vi "Dipper Fridge Resistance Measurement 1.0.vi"() -> ()   [LabVIEW 2011]
uses:
  <vilib>/express/express arith-compare/Formula/XNode/ExpressFormulaBlockNode.xnode
panel:
  out "Heater Power (%)":string
  in  "Save":bool
  out "var":i32
  in  "error in (no error) 2":errorcluster
  in  "Output Range":string(combo)
  in  "Heater Power (%)":dbl caption="y"
  out "Heater Type (in Ohm)":string
  out "Heater Current (in %)":string
  out "Heater":bool
  in  "Heater":bool
  out "x+y":dbl
  out "Boolean":bool
  in  "Power":bool
  in  "Date format (0)":enum16{"short", "long", "abbreviated"}(ring)
  out "Lakeshore":cluster{dbl[], dbl[unit][]}(graph)
  out "Chanel B":cluster{dbl[], dbl[unit][]}(graph)
  out "size (in bytes)":i64
  out "Chanel A":cluster{dbl[], dbl[]}(graph)
  out "Warning":string="Can't be smaller than 1 s"
  in  "File Path":path
  out "current time":timestamp
  out "Number of Data points":i32
  in  "Time delay":u32
  in  "error in (no error)":errorcluster
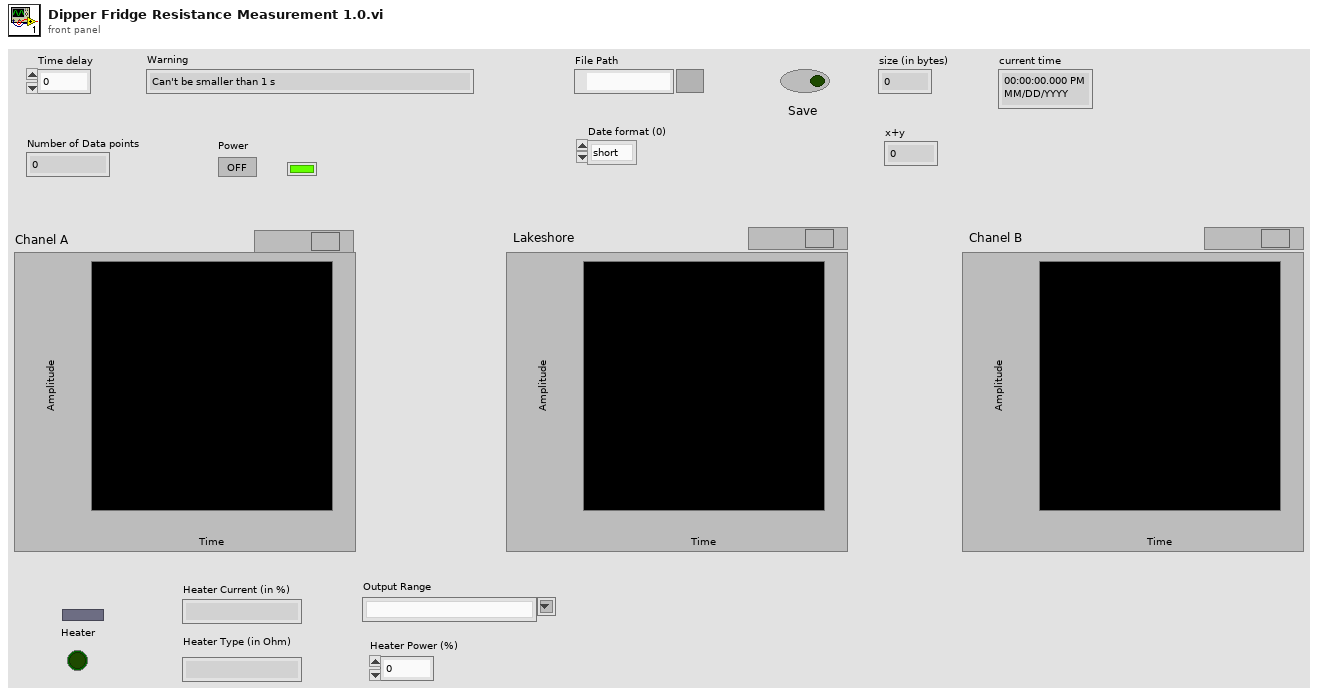
[diagram p1: front panel]
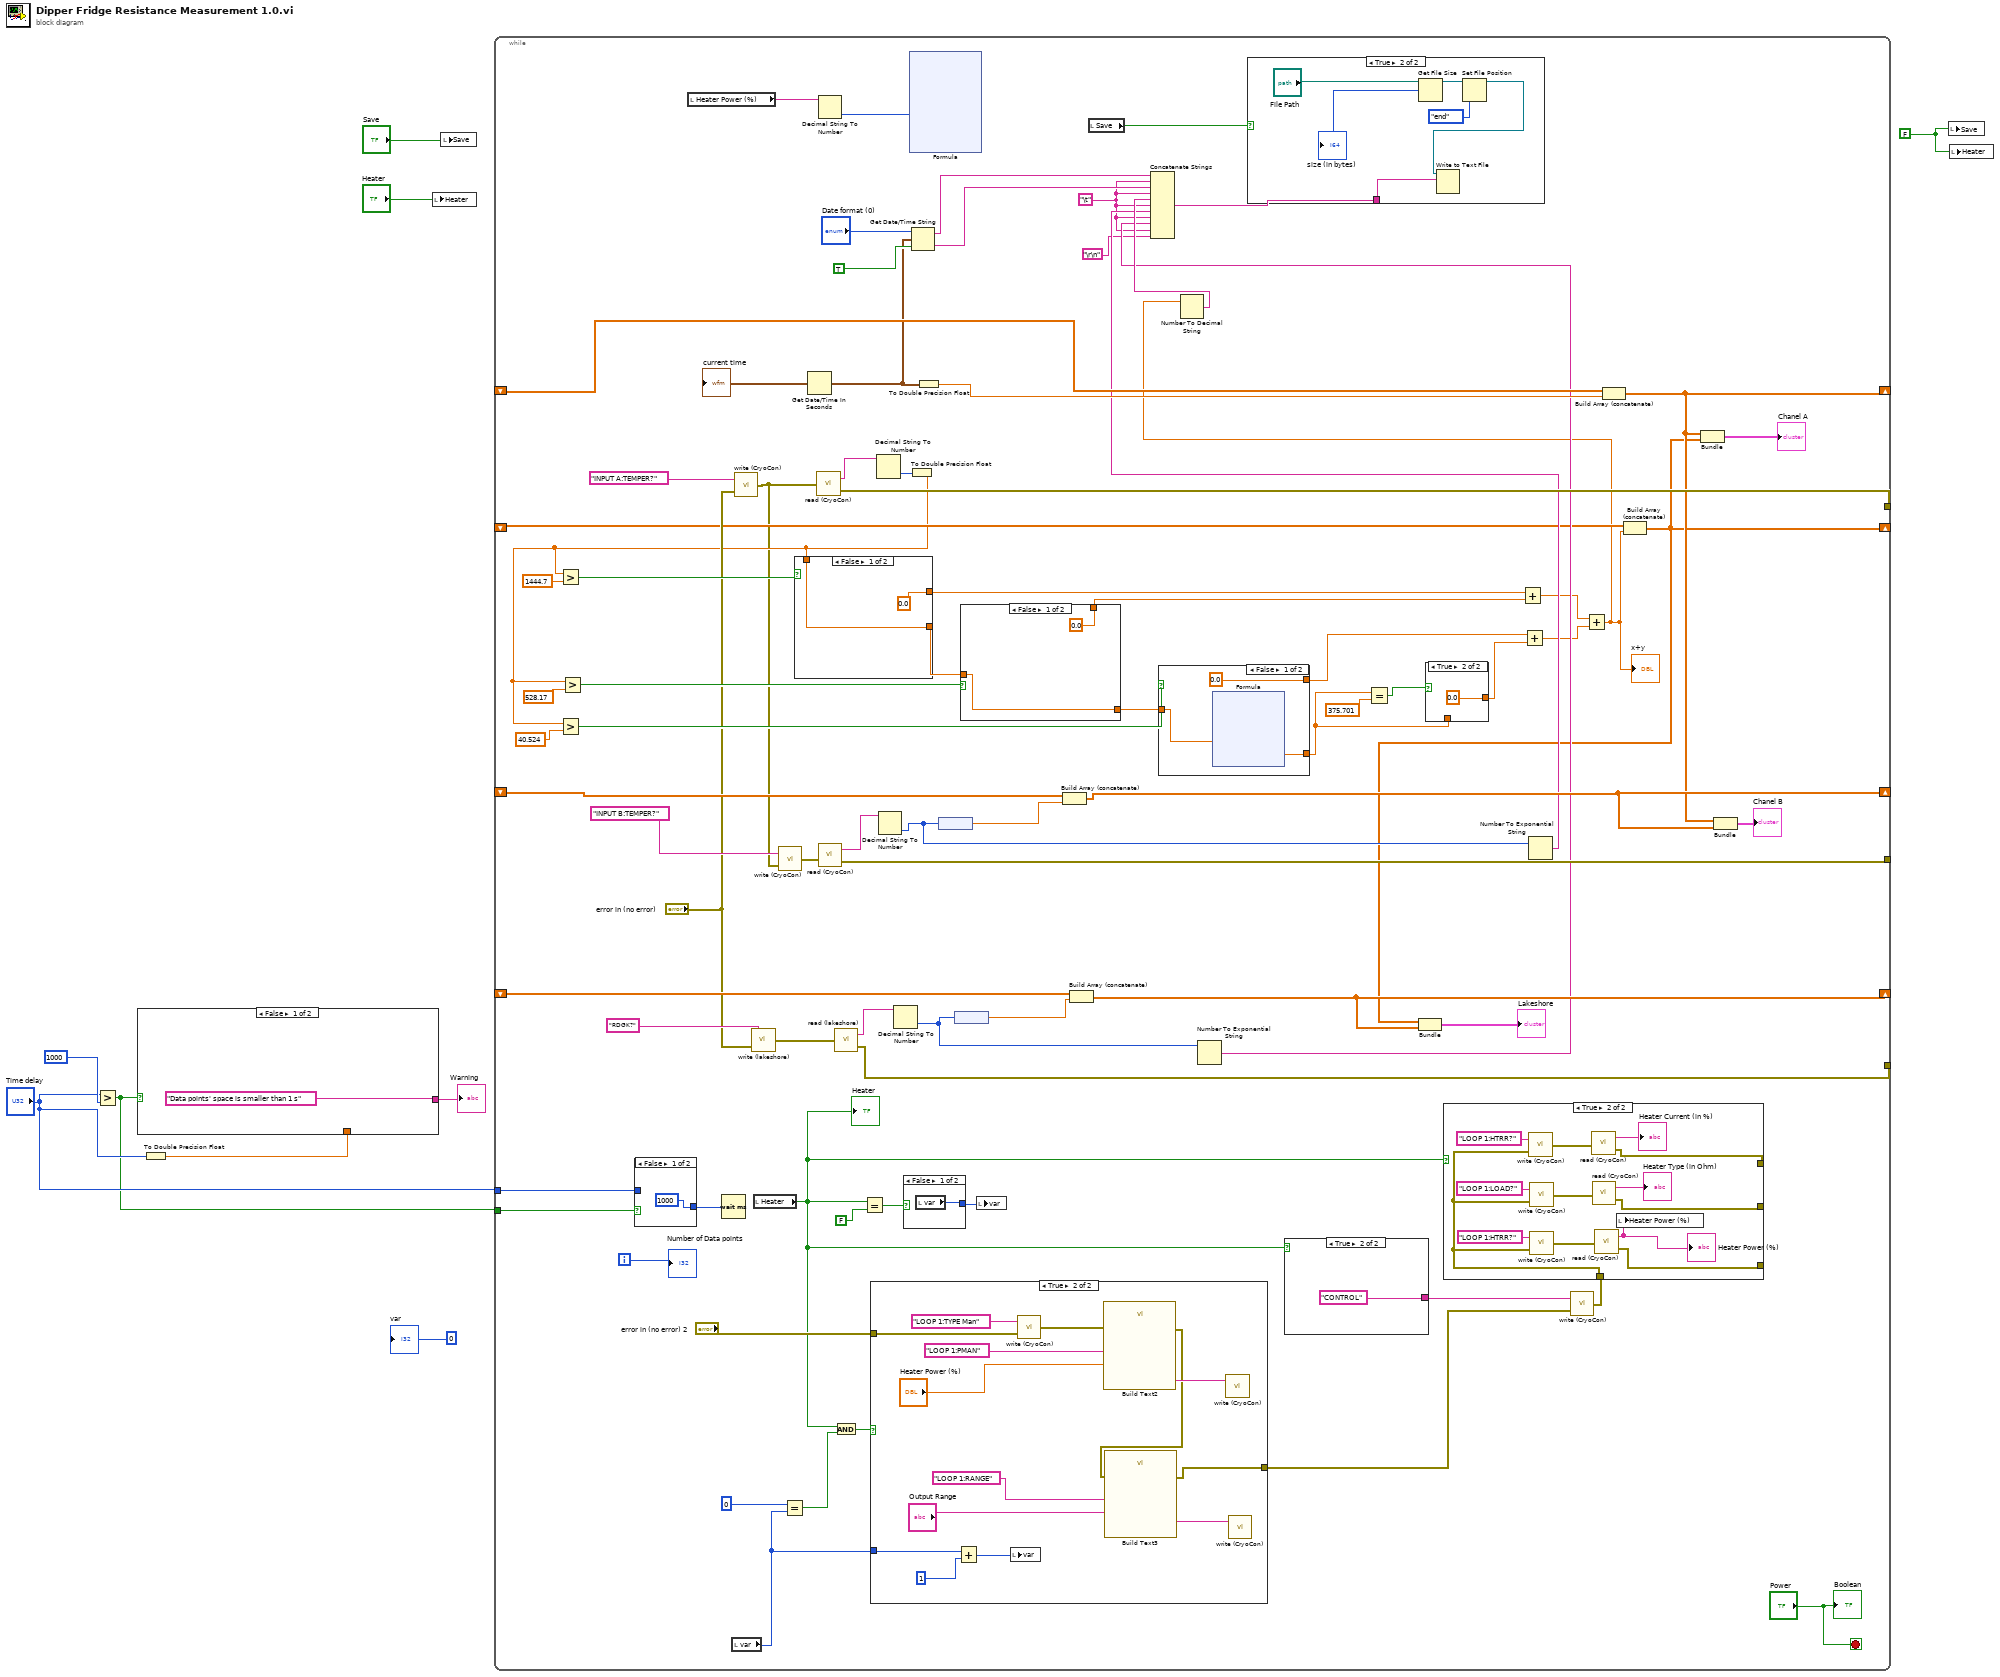
[diagram p0: block diagram]
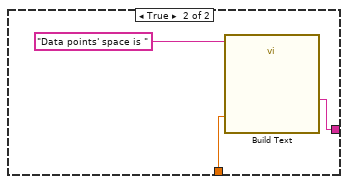
[diagram p2: hidden frame]
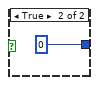
[diagram p3: hidden frame]
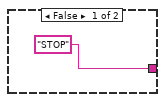
[diagram p6: hidden frame]
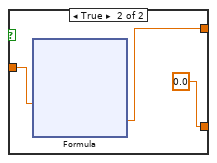
[diagram p8: hidden frame]
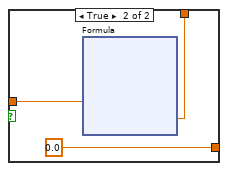
[diagram p9: hidden frame]
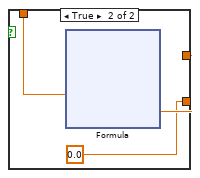
[diagram p10: hidden frame]
diagram:
  w2 = FALSE ("Save")
  n1 = Greater?(x="Time delay", y=u32 1000 ("x")) -> (0:w5:bool)
  n2 = To Double Precision Float(number="Time delay") -> (double precision float=w9:dbl)
  n3 = case shown="False" w5 {
    tunnel: w9 -> [_ w11]
    tunnel: ["Data points' space is smaller than 1 s" w13] -> w8
    frame False {
    }
    frame True {
      n4 = call "Build Text"("Beginning Text"="Data points' space is ", "Y"=w11) -> ("Result"=w13:string)  [unwired: 12 in, 1 out]
    }
  }
  "Warning" <- w8
  n5 = local write "Heater"("Heater") -> ()
  n6 = local write "Save"("Save") -> ()
  n7 = while {
    tunnel: [w90] -> _
    tunnel: [w89] -> _
    tunnel: [w85] -> _
    shift-right: [w66] -> _
    shift-left: _ -> [w80]
    tunnel: "Time delay" -> [w79]
    tunnel: w5 -> [w78]
    shift-right: [w70] -> _
    shift-left: _ -> [w71]
    shift-right: [w67] -> _
    shift-left: _ -> [w68]
    shift-right: [w45] -> _
    shift-left: _ -> [w48]
    i -> [w82]
    stop <- "Power" stop-if-true
    w22 = "\t"
    n8 = case shown="False" w78 {
      tunnel: w79 -> [_ w190]
      tunnel: [1000 w190] -> w77
      frame False {
      }
      frame True {
      }
    }
    n9 = local read "Heater Power (%)"() -> (w21:string)
    n10 = Wait (ms)(milliseconds to wait=w77) -> ()  [unwired: 1 out]
    n11 = local read "var"() -> (w28:i32)
    n12 = call "write (CryoCon).vi"("error in (no error)"="error in (no error)", "write buffer"="INPUT A:TEMPER?") -> ("error out"=w14:errorcluster)
    n13 = call "write (lakeshore).vi"("error in (no error)"="error in (no error)", "write buffer"="RDGK?") -> ("error out"=w84:errorcluster)
    n14 = local read "Heater"() -> (w15:bool)
    "Heater" <- w15
    n15 = call "write (CryoCon).vi"("error in (no error)"=w14, "write buffer"="INPUT B:TEMPER?") -> ("error out"=w91:errorcluster)
    n16 = Equal?(x=0, y=w28) -> (x = y?=w26:bool)
    n17 = Get Date/Time In Seconds() -> (seconds since 1Jan1904=w76:timestamp)
    "current time" <- w76
    n18 = call "read (CryoCon).vi"("error in (no error)"=w14) -> ("read buffer"=w87:string, "error out"=w89:errorcluster)
    n19 = Decimal String To Number(string=w21) -> (number=w20:i32)  [unwired: 2 in, 1 out]
    n20 = call "read (CryoCon).vi"("error in (no error)"=w91) -> ("read buffer"=w88:string, "error out"=w90:errorcluster)
    n21 = call "read (lakeshore).vi"("error in (no error)"=w84) -> ("read buffer"=w86:string, "error out"=w85:errorcluster)
    n22 = And(x=w15, y=w26) -> (x .and. y?=w25:bool)
    n23 = Equal?(x=w15, y=FALSE ("Heater")) -> (x = y?=w17:bool)
    n24 = case shown="True" w25 {
      tunnel: [w108 w116] -> w24
      tunnel: "error in (no error) 2" -> [w108 w112]
      tunnel: w28 -> [_ w115]
      frame False {
      }
      frame True {
        n25 = Add(x=w115, y=1) -> (x+y=w113:i32)
        n26 = local write "var"(w113) -> ()
        n27 = call "write (CryoCon).vi"("error in (no error)"=w112, "write buffer"="LOOP 1:TYPE Man") -> ("error out"=w111:errorcluster)
        n28 = call "Build Text2"("x"="LOOP 1:PMAN" ("write buffer"), "y"="Heater Power (%)", "error in (no error)"=w111) -> ("Result"=w121:string, "error out"=w117:errorcluster)  [unwired: 11 in]
        n29 = call "Build Text3"("x"="LOOP 1:RANGE" ("write buffer"), "y"="Output Range", "error in (no error)"=w117) -> ("Result"=w118:string, "error out"=w116:errorcluster)  [unwired: 11 in]
        n30 = call "write (CryoCon).vi"("write buffer"=w121) -> ()  [unwired: 1 in, 1 out]
        n31 = call "write (CryoCon).vi"("write buffer"=w118) -> ()  [unwired: 1 in, 1 out]
      }
    }
    n32 = Decimal String To Number(string=w87) -> (number=w74:i32)  [unwired: 2 in, 1 out]
    n33 = Decimal String To Number(string=w88) -> (number=w64:i32)  [unwired: 2 in, 1 out]
    n34 = Decimal String To Number(string=w86) -> (number=w63:i32)  [unwired: 2 in, 1 out]
    n35 = case shown="False" w17 {
      tunnel: [w94 0] -> w16
      frame False {
        n36 = local read "var"() -> (w94:i32)
      }
      frame True {
      }
    }
    n37 = xnode "Formula"("X1"=w20) -> ()  [unwired: 3 in, 2 out]
    n38 = To Double Precision Float(number=w74) -> (double precision float=w37:dbl)
    n39 = Greater?(x=w37, y=1444.7) -> (0:w56:bool)
    n40 = Greater?(x=w37, y=40.524) -> (0:w53:bool)
    n41 = Greater?(x=w37, y=528.17) -> (0:w55:bool)
    n42 = case shown="False" w56 {
      tunnel: w37 -> [w176 w180]
      tunnel: [0.0 w179] -> w42
      tunnel: [w176 0.0] -> w39
      frame False {
      }
      frame True {
        n43 = xnode "Formula"("X1"=w180) -> ("Result"=w179:dbl)  [unwired: 1 in, 1 out]
      }
    }
    n44 = Get Date/Time String(date format (0)="Date format (0)", seconds (now)=w76, want seconds? (F)=TRUE) -> (date string=w62:string, time string=w61:string)
    n45 = To Double Precision Float(number=w76) -> (double precision float=w75:dbl)
    n46 = node(w64) -> (w72:dbl[unit])
    n47 = node(w63) -> (w47:dbl[unit])
    n48 = case shown="False" w55 {
      tunnel: [0.0 w167] -> w41
      tunnel: w39 -> [w163 w166]
      tunnel: [w163 0.0] -> w38
      frame False {
      }
      frame True {
        n49 = xnode "Formula"("X2"=w166) -> ("Result"=w167:dbl)  [unwired: 1 in, 1 out]
      }
    }
    n50 = local write "var"(w16) -> ()
    n51 = Build Array (concatenate)(w71, w72) -> (w70:dbl[unit][])
    n52 = Build Array (concatenate)(w68, w47) -> (w67:dbl[unit][])
    n53 = local read "Save"() -> (w23:bool)
    n54 = case shown="False" w53 {
      tunnel: [0.0 w154] -> w40
      tunnel: [w142 0.0] -> w33
      tunnel: w38 -> [w141 w152]
      frame False {
        n55 = xnode "Formula"("X4"=w141) -> ("Result"=w142:dbl)  [unwired: 1 in, 1 out]
      }
      frame True {
        n56 = xnode "Formula"("X3"=w152) -> ("Result"=w154:dbl)  [unwired: 1 in, 1 out]
      }
    }
    n57 = Number To Exponential String(number=w63) -> (E-format string=w58:string)  [unwired: 3 in]
    n58 = case shown="True" w15 {
      tunnel: ["STOP" ("write buffer") "CONTROL" ("write buffer")] -> w31
      frame False {
      }
      frame True {
      }
    }
    n59 = Equal?(x=w33, y=375.701) -> (x = y?=w36:bool)
    n60 = case shown="True" w36 {
      tunnel: [w139 0.0 ("y")] -> w34
      tunnel: w33 -> [w139 _]
      frame False {
      }
      frame True {
      }
    }
    n61 = Add(x=w42, y=w41) -> (x+y=w50:dbl)
    n62 = Add(x=w40, y=w34) -> (x+y=w49:dbl)
    n63 = Number To Exponential String(number=w64) -> (E-format string=w59:string)  [unwired: 3 in]
    n64 = call "write (CryoCon).vi"("error in (no error)"=w24, "write buffer"=w31) -> ("error out"=w30:errorcluster)
    n65 = case shown="True" w15 {
      tunnel: [w123 w130] -> _
      tunnel: [w123 w129] -> _
      tunnel: w30 -> [w123 w128]
      tunnel: [w123 w127] -> _
      frame False {
      }
      frame True {
        n66 = call "write (CryoCon).vi"("error in (no error)"=w128, "write buffer"="LOOP 1:HTRR?") -> ("error out"=w136:errorcluster)
        n67 = call "write (CryoCon).vi"("error in (no error)"=w128, "write buffer"="LOOP 1:LOAD?") -> ("error out"=w133:errorcluster)
        n68 = call "write (CryoCon).vi"("error in (no error)"=w128, "write buffer"="LOOP 1:HTRR?") -> ("error out"=w126:errorcluster)
        n69 = call "read (CryoCon).vi"("error in (no error)"=w136) -> ("read buffer"=→"Heater Current (in %)":string, "error out"=w130:errorcluster)
        n70 = call "read (CryoCon).vi"("error in (no error)"=w133) -> ("read buffer"=→"Heater Type (in Ohm)":string, "error out"=w129:errorcluster)
        n71 = call "read (CryoCon).vi"("error in (no error)"=w126) -> ("read buffer"=w124:string, "error out"=w127:errorcluster)
        "Heater Power (%)" <- w124
        n72 = local write "Heater Power (%)"(w124) -> ()
      }
    }
    n73 = Add(x=w50, y=w49) -> (x+y=w32:dbl)
    "x+y" <- w32
    n74 = Number To Decimal String(number=w32) -> (decimal integer string=w60:string)  [unwired: 1 in]
    n75 = Concatenate Strings(w62, w22, w61, w22, w60, w22, w59, w22, w58, w22, "\r\n") -> (w73:string)
    n76 = case shown="True" w23 {
      tunnel: w73 -> [_ w196]
      frame False {
      }
      frame True {
        n77 = Get File Size(file="File Path") -> (refnum out=w194:refnum<file>, size (in bytes)=→"size (in bytes)":i64)  [unwired: 1 in, 1 out]
        n78 = Set File Position(refnum=w194, from (0:start)=enum16{"start", "end", "current"}."end") -> (refnum out=w193:refnum<file>)  [unwired: 2 in, 1 out]
        n79 = Write to Text File(file (use dialog)=w193, text=w196) -> ()  [unwired: 2 in, 3 out]
      }
    }
    n80 = Build Array (concatenate)(w80, w75) -> (w66:dbl[])
    n81 = Build Array (concatenate)(w48, w32) -> (w45:dbl[])
    n82 = Bundle(w45, w67) -> (→"Lakeshore":cluster{dbl[], dbl[unit][]})  [unwired: 1 in]
    n83 = Bundle(w66, w45) -> (→"Chanel A":cluster{dbl[], dbl[]})  [unwired: 1 in]
    n84 = Bundle(w66, w70) -> (→"Chanel B":cluster{dbl[], dbl[unit][]})  [unwired: 1 in]
    "Number of Data points" <- w82
    "Boolean" <- "Power"
  }
  n85 = local write "Save"(w2) -> ()
  n86 = local write "Heater"(w2) -> ()
  "var" <- 0 ("var")
